vi "Read Restore Point.vi"(11 "Test Step Dialog in":refnum<class "Test Step Dialog.lvclass">) -> (2 "Restore Point":bool, 3 "Test Step Dialog out":refnum<class "Test Step Dialog.lvclass">)   [LabVIEW 2017, in "Test Step Dialog.lvclass"]
uses:
  <vilib>/gpm_packages/@cs/Test-executive-builder/Source/Test Executive Builder Dialogs/Test Step Dialog/Test Step Dialog.lvclass
  <vilib>/gpm_packages/@cs/Test-executive-builder/Source/Test Executive Builder Dialogs/Test Step Dialog/Test Step Dialog.lvclass/Test Step Dialog.ctl
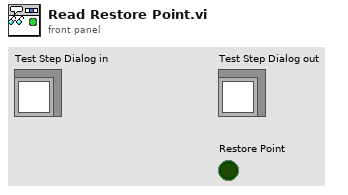
[diagram p1: front panel]
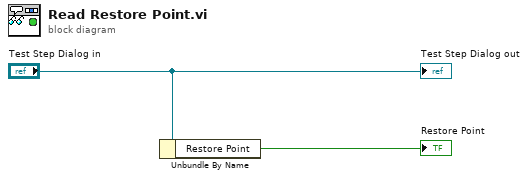
[diagram p0: block diagram]
diagram:
  n1 = Unbundle By Name("Test Step Dialog in") -> ("Restore Point"=→"Restore Point":bool)
  "Test Step Dialog out" <- "Test Step Dialog in"
